vi "Init Hardware.vi"(8 "error in (no error)":errorcluster, 11 "Andeen-Hagerling Driver in":refnum<class "Andeen-Hagerling Driver.lvclass">) -> (0 "error out":errorcluster, 3 "Andeen-Hagerling Driver out":refnum<class "Andeen-Hagerling Driver.lvclass">)   [LabVIEW 2019, in "Andeen-Hagerling Driver.lvclass"]
uses:
  Andeen-Hagerling Driver.lvclass
  C:/GitHub/NHMFL_Core/Libraries/Instruments/Instrument Driver/Instrument Driver.lvclass
  Instrument Driver/Instrument Driver.lvclass/Instrument Driver.ctl
  Instrument Driver/Read Recorder name.vi
  Instrument Driver/Write Channel names.vi
  Instrument Driver/Write Channel units.vi
  Simple VISA Reader/Simple VISA Reader Driver.lvclass
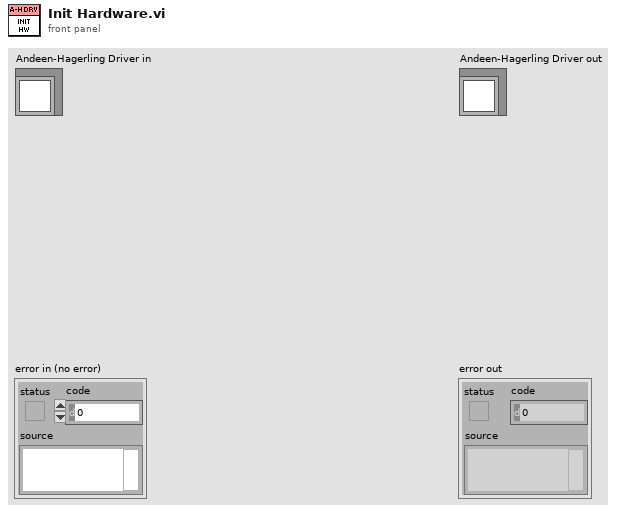
[diagram p1: front panel]
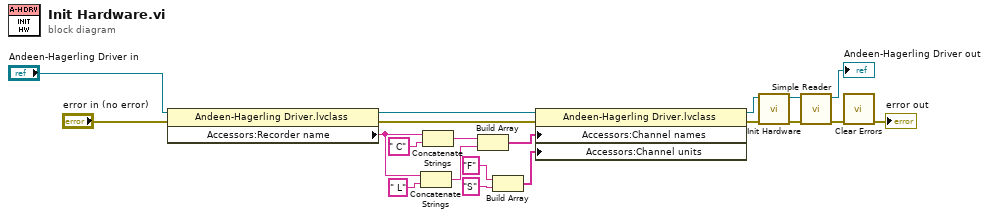
[diagram p0: block diagram]
diagram:
  n1 = property class="Andeen-Hagerling Driver.lvclass"(reference="Andeen-Hagerling Driver in", error in="error in (no error)") -> (reference out=w12:refnum<class "Andeen-Hagerling Driver.lvclass">, error out=w11:errorcluster, "Accessors:Recorder name"=w17:string)
  n2 = Concatenate Strings(w17, " L") -> (w19:string)
  n3 = Concatenate Strings(w17, " C") -> (w16:string)
  n4 = Build Array(w16, w19) -> (w14:string[])
  n5 = Build Array("F", "S" ("element")) -> (w13:string[])
  n6 = property class="Andeen-Hagerling Driver.lvclass"(reference=w12, error in=w11, "Accessors:Channel names"=w14, "Accessors:Channel units"=w13) -> (reference out=w9:refnum<class "Andeen-Hagerling Driver.lvclass">, error out=w7:errorcluster)
  n7 = call-parent "Init Hardware.vi"("error in (no error)"=w7, "Instrument Driver in"=w9) -> ("error out"=w3:errorcluster, "Instrument Driver out"=w5:refnum<class "Andeen-Hagerling Driver.lvclass">)  [unwired: 8 in]
  n8 = call-dynamic "Simple Reader.vi"("error in (no error)"=w3, "Andeen-Hagerling Driver in"=w5) -> ("error out"=w2:errorcluster, "Andeen-Hagerling Driver out"=→"Andeen-Hagerling Driver out":refnum<class "Andeen-Hagerling Driver.lvclass">)  [unwired: 7 in, 1 out]
  n9 = call <vilib>:"Clear Errors.vi"("error in (no error)"=w2) -> ("error out"=→"error out":errorcluster)  [unwired: 5 in, 1 out]
